vi "mainStationMeteo_version_avec_cluster_non_testé.vi"() -> ()   [LabVIEW 2017]
doc: "Le projet station météo, permet de relevées les informations des capteurs suivant:\n Température\n Girouette\n Anémomètre\n Pluviométrie\n Humidité\n Luminosité\n\nIl suffit de choisir un intervalle de mesure sur la command en haut à gauche\net de lancer l'acquisition (Bouton acquisition), si des alarmes existent, elles seront enregistrées sur le fichier alarmes.txt du même dossier.\n Pour arrêter ou recommencer l'acquisition, cliquer sur le bouton Stop/Initialisation deux fois puis relancer l'acquisition."
panel:
  out "Lecture du fichier":string
  out "sortie d'erreur":errorcluster caption="CLUSTER d'erreur"
  in  "Choix intervale de mesure":dbl caption="Définir l'intervale d'acquisition (s)"
  out "Valeurs en temps réel":string
  in  "Acquisition":bool
  out "Alarme":bool
  out "Etat":T1(ring)
  in  "Stop/Initialisation":bool
  # "Station Météo"
  # "BENOIT MANGEARD | JIXIONG LIU - 2018"
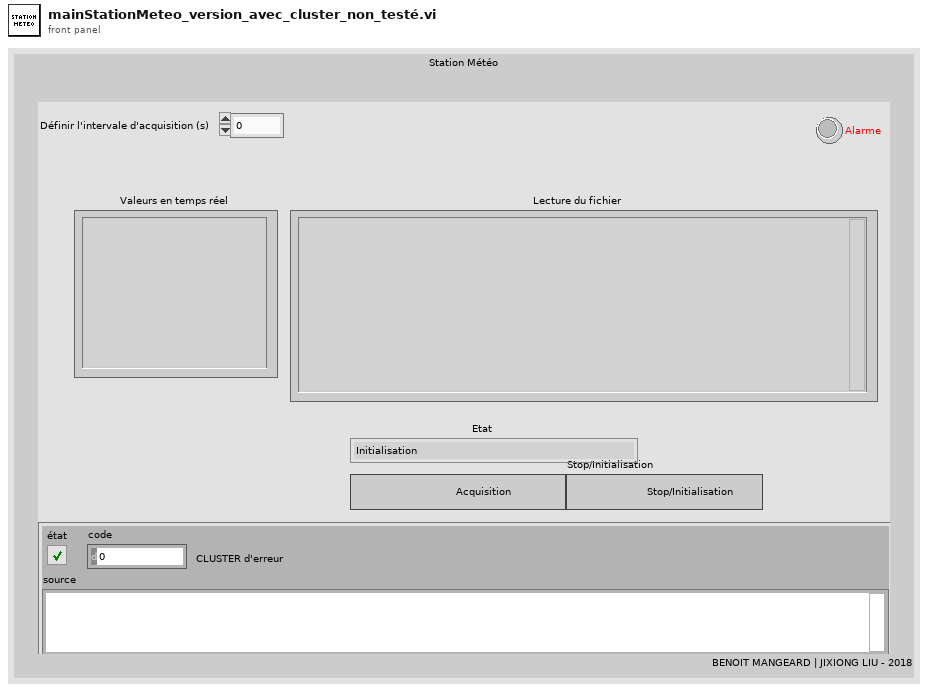
[diagram p1: front panel]
types:
  T1 = enum16{"Initialisation", "Acquisition", "Analyse", "Enregistrer", "Vérification du temps et Stop", "Fin"}
  T2 = cluster{"Température":dbl, "Vent":dbl, "Chaîne":string, dbl, u32}
  T3 = cluster{"Chaîne":string, "Chaîne":string, "Chaîne":string}
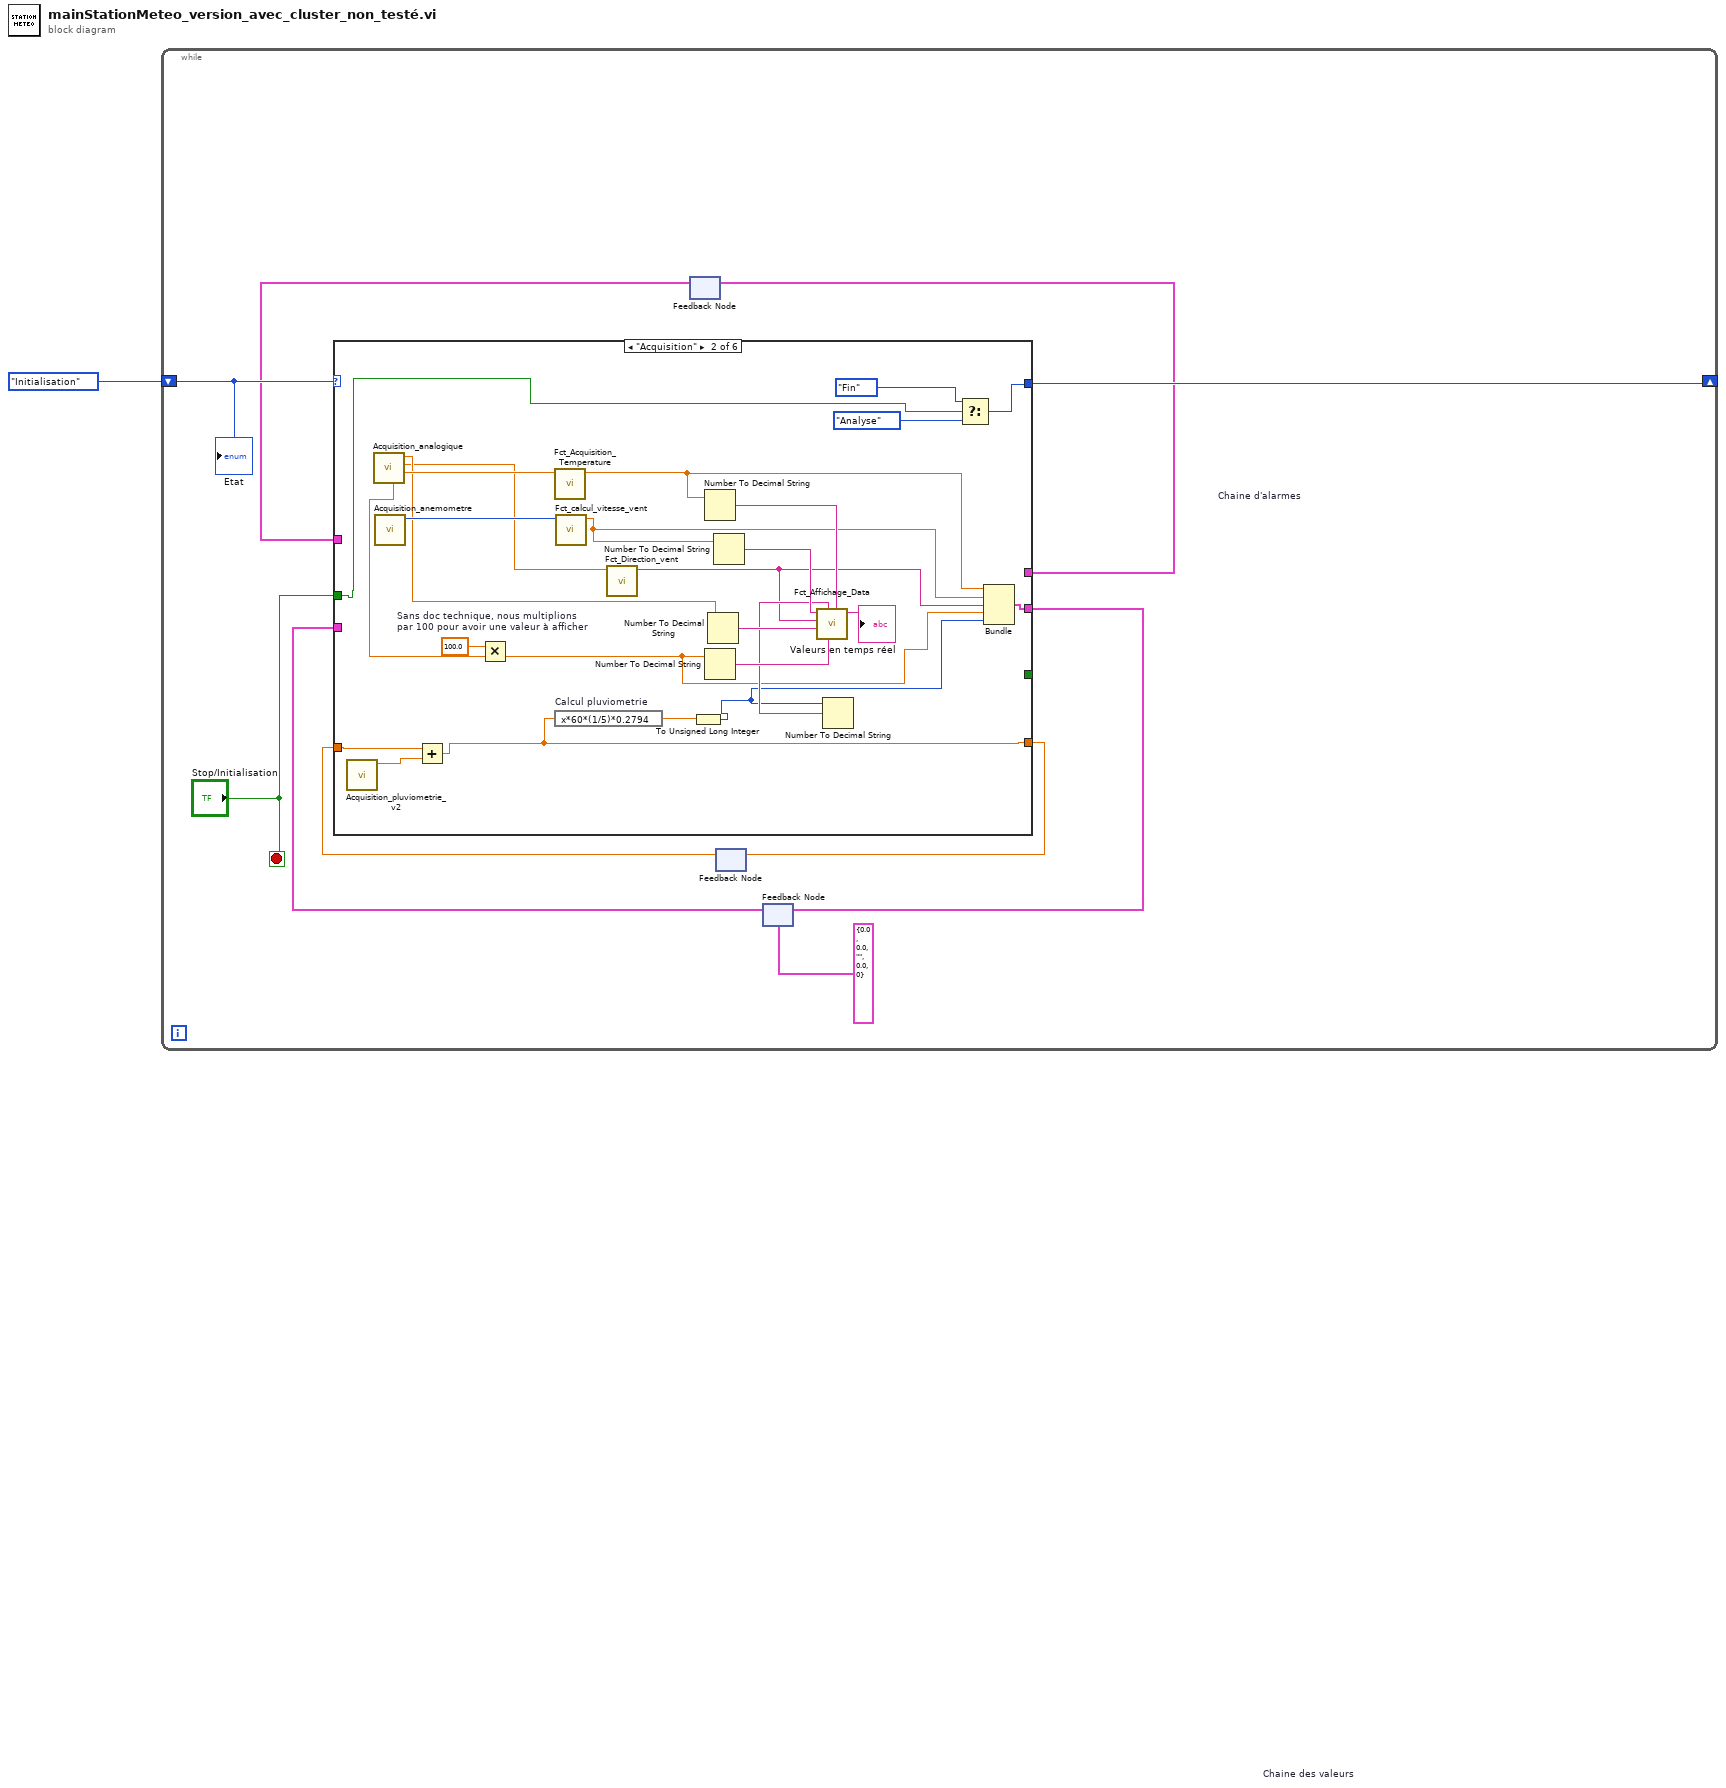
[diagram p0: block diagram]
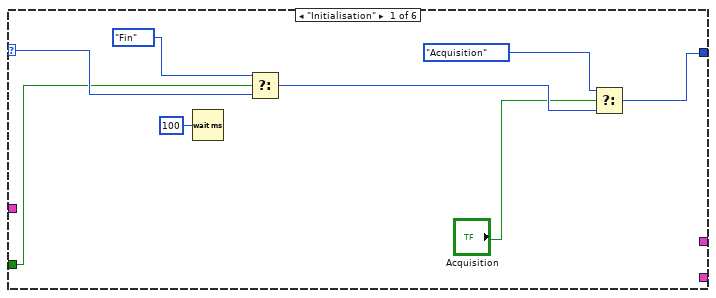
[diagram p2: hidden frame]
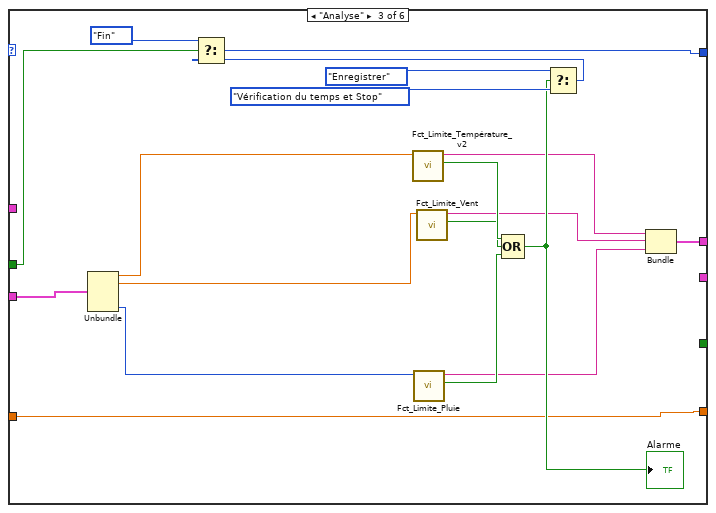
[diagram p3: hidden frame]
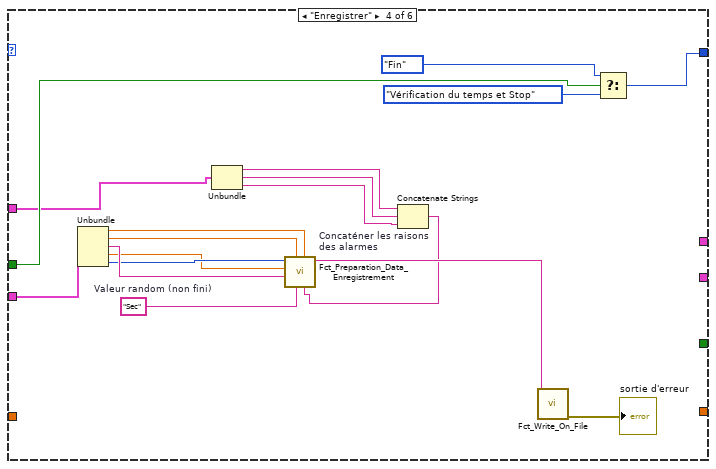
[diagram p4: hidden frame]
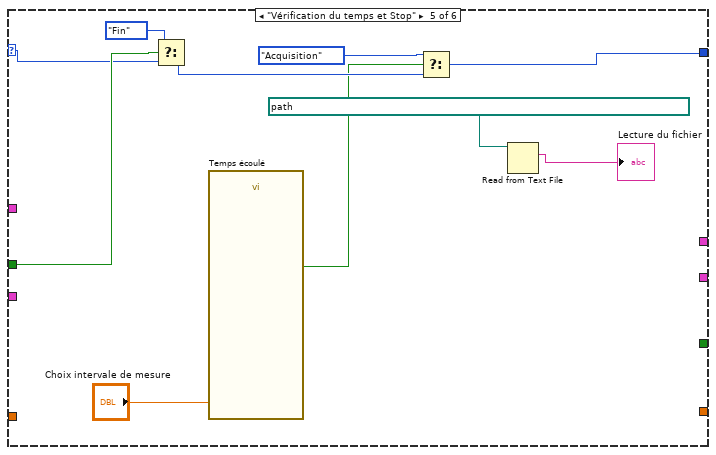
[diagram p5: hidden frame]
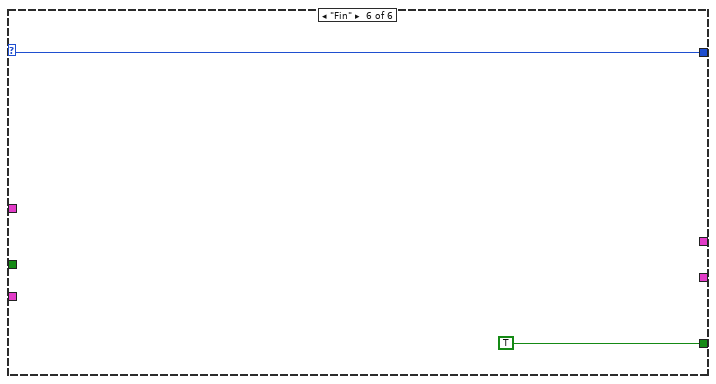
[diagram p6: hidden frame]
diagram:
  n1 = while {
    shift-right: [w11] -> _
    shift-left: T1."Initialisation" -> [w10]
    stop <- "Stop/Initialisation" stop-if-true
    n2 = feedback #1 "Chaine d'alarmes"() -> (w2:T3)  [unwired: 1 in]
    n3 = feedback #2() -> (w6:dbl)  [unwired: 1 in]
    n4 = feedback #3 "Chaine des valeurs"(T2 {"Température"=0.0, "Vent"=0.0, "Chaîne"="", 0.0, 0}) -> (w8:T2)
    n5 = case "Structure Condition" shown="\"Acquisition\"" w10 {
      selector: w10 -> [w18 _ _ _ w86 w94]
      tunnel: [w14 w33 w56 w78 w92 w94] -> w11
      tunnel: "Stop/Initialisation" -> [w12 w29 w58 w76 w89 _]
      tunnel: [_ _ _ _ _ TRUE] -> _
      tunnel: [_ w22 _ _ _ _] -> w5
      tunnel: w8 -> [_ _ w54 w74 _ _]
      tunnel: [_ w21 w50 _ _ _] -> w7
      tunnel: w6 -> [_ w20 w50 _ _ _]
      tunnel: [_ _ w46 _ _ _] -> w3
      tunnel: w2 -> [_ _ _ w68 _ _]
      frame "Initialisation" {
        n6 = Wait (ms)(milliseconds to wait=u32 100 ("attente (ms)")) -> ()  [unwired: 1 out]
        n7 = Select(t=T1."Fin", s=w12, f=w18) -> (s? t:f=w16:T1)
        n8 = Select(t=T1."Acquisition", s="Acquisition", f=w16) -> (s? t:f=w14:T1)
      }
      frame "Acquisition" {
        w36 = 100.0  # Sans doc technique, nous multiplions  par 100 pour avoir une valeur à afficher
        n9 = call "Acquisition_pluviometrie_v2.vi"() -> ("Numérique"=w40:dbl)  [unwired: 11 in]
        n10 = call "Acquisition_analogique.vi"() -> ("Température"=w43:dbl, "Girouette"=w28:dbl, "Humidité"=w35:dbl, "Lumière"=w39:dbl)  [unwired: 8 in]
        n11 = call "Acquisition_anemometre.vi"() -> ("data"=w41:u32)  [unwired: 11 in]
        n12 = Add(x=w20, y=w40) -> (x+y=w21:dbl)
        n13 = Multiply(x=w36, y=w39) -> (x*y=w24:dbl)
        n14 = call "Fct_Acquisition_Temperature.vi"("Tension"=w43) -> ("Température"=w27:dbl)  [unwired: 7 in, 3 out]
        n15 = expression code="x*60*(1/5)*0.2794" "Calcul pluviometrie"(w21) -> (w34:dbl)
        n16 = call "Fct_calcul_vitesse_vent.vi"("data"=w41) -> ("Vent"=w26:dbl)  [unwired: 10 in]
        n17 = call "Fct_Direction_vent.vi"("Tension Girouette"=w28) -> ("Chaîne"=w25:string)  [unwired: 10 in]
        n18 = To Unsigned Long Integer(number=w34) -> (unsigned 32bit integer=w23:u32)
        n19 = Number To Decimal String(number=w27) -> (decimal integer string=w44:string)  [unwired: 1 in]
        n20 = Number To Decimal String(number=w24) -> (decimal integer string=w38:string)  [unwired: 1 in]
        n21 = Number To Decimal String(number=w35) -> (decimal integer string=w37:string)  [unwired: 1 in]
        n22 = Number To Decimal String(number=w26) -> (decimal integer string=w42:string)  [unwired: 1 in]
        n23 = Number To Decimal String(number=w23) -> (decimal integer string=w30:string)  [unwired: 1 in]
        n24 = call "Fct_Affichage_Data.vi"("Température"=w44, "Luminosité"=w38, "Pluiviométrie"=w30, "Humidité"=w37, "Direction du vent"=w25, "Vitesse vent"=w42) -> ("Sortie"=→"Valeurs en temps réel":string)  [unwired: 5 in]
        n25 = Select(t=T1."Fin", s=w29, f=T1."Analyse") -> (s? t:f=w33:T1)
        n26 = Bundle("Température"=w27, "Vent"=w26, "Chaîne"=w25, w24, w23) -> (w22:T2)  [unwired: 1 in]
      }
      frame "Analyse" {
        n27 = Unbundle(w54) -> ("Température"=w53:dbl, "Vent"=w52:dbl, w51:u32)  [unwired: 2 out]
        n28 = call "Fct_Limite_Température_v2.vi"("Température"=w53) -> ("Booléen"=w62:bool, "Chaîne"=w49:string)  [unwired: 9 in]
        n29 = call "Fct_Limite_Pluie.vi"("Pluie"=w51) -> ("Booléen"=w60:bool, "Chaîne"=w47:string)  [unwired: 9 in]
        n30 = call "Fct_Limite_Vent.vi"("Vent"=w52) -> ("Booléen"=w61:bool, "Chaîne"=w48:string)  [unwired: 9 in]
        n31 = Compound Arithmetic op=OR ("Opérateur arithmétique")(w62, w61, w60) -> (w59:bool)
        "Alarme" <- w59
        n32 = Select(t=T1."Enregistrer", s=w59, f=T1."Vérification du temps et Stop") -> (s? t:f=w55:T1)
        n33 = Select(t=T1."Fin", s=w58, f=w55) -> (s? t:f=w56:T1)
        n34 = Bundle("Chaîne"=w49, "Chaîne"=w48, "Chaîne"=w47) -> (w46:T3)  [unwired: 1 in]
      }
      frame "Enregistrer" {
        w80 = "Sec"  # Valeur random (non fini)
        n35 = Unbundle(w74) -> ("Température"=w73:dbl, "Vent"=w72:dbl, "Chaîne"=w71:string, w69:dbl, w70:u32)
        n36 = Unbundle(w68) -> ("Chaîne"=w65:string, "Chaîne"=w67:string, "Chaîne"=w66:string)
        n37 = Concatenate Strings "Concaténer les raisons des alarmes"(w65, w67, w66) -> (w79:string)
        n38 = call "Fct_Preparation_Data_Enregistrement.vi"("Motif"=w79, "Temperature"=w73, "Humidité"=w80, "Vitesse vent"=w72, "Direction Vent"=w71, "Luminosité"=w69, "Précipitation"=w70) -> ("Chaîne"=w81:string)  [unwired: 4 in]
        n39 = call "Fct_Write_On_File.vi"("Chaîne"=w81) -> ("sortie d'erreur"=→"sortie d'erreur":errorcluster)  [unwired: 10 in]
        n40 = Select(t=T1."Fin", s=w76, f=T1."Vérification du temps et Stop") -> (s? t:f=w78:T1)
      }
      frame "Vérification du temps et Stop" {
        n41 = Select(t=T1."Fin", s=w89, f=w86) -> (s? t:f=w87:T1)
        n42 = call "Temps écoulé"("Time Target (s)"="Choix intervale de mesure") -> ("Time has Elapsed"=w85:bool)  [unwired: 11 in, 7 out]
        n43 = Select(t=T1."Acquisition", s=w85, f=w87) -> (s? t:f=w92:T1)
        n44 = Read from Text File(file (use dialog)=path "E:/ESIGELEC/Phase 2/Instrumentation et systèmes/Station_meteo/Alarmes.txt" ("fichier (utiliser une boîte de dialogue)")) -> (text=→"Lecture du fichier":string)  [unwired: 3 in, 3 out]
      }
      frame "Fin" {
      }
    }
    n45 = feedback-in #1(w3) -> ()
    n46 = feedback-in #2(w7) -> ()
    n47 = feedback-in #3(w5) -> ()
    "Etat" <- w10
  }
